vi "Prototype.vi"(8 "error in (no error)":errorcluster, 10 "Target Method Prototyper in":refnum<class "Target Method Icon Reader.lvclass">, 11 "Scripter in":refnum<class "Message Scripter.lvclass">) -> (0 "error out":errorcluster, 2 "Target Method Prototyper out":refnum<class "Target Method Icon Reader.lvclass">, 3 "Scripter out":refnum<class "Message Scripter.lvclass">)   [LabVIEW 2020, in "Message Maker.lvlib" / "Target Method Icon Reader.lvclass"]
uses:
  Target Method Icon Reader.lvclass
  Message Scripter/Message Scripter.lvclass
  Message Maker.lvlib
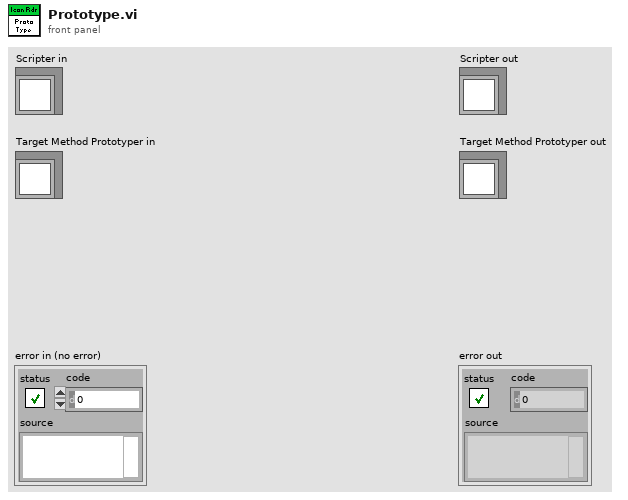
[diagram p1: front panel]
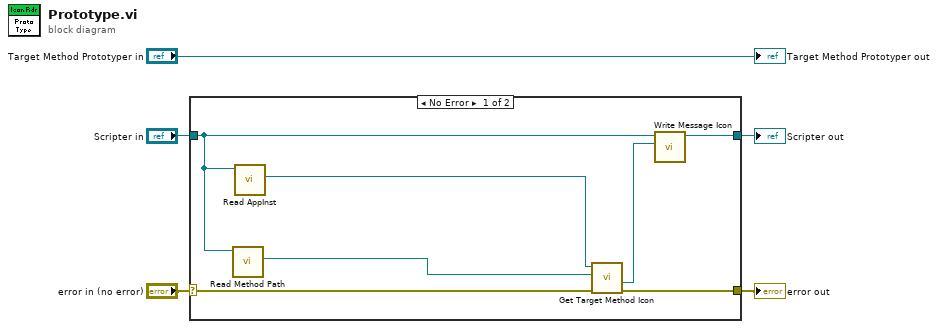
[diagram p0: block diagram]
diagram:
  n1 = case shown="No Error" "error in (no error)" {
    selector: "error in (no error)" -> [w12 w13]
    tunnel: "Scripter in" -> [w11 w14]
    tunnel: [w8 w14] -> w3
    tunnel: [w10 w13] -> w1
    frame No Error {
      n2 = call "Read Method Path.vi"("Message Maker in"=w11) -> ("Method Path"=w6:path)  [unwired: 10 in]
      n3 = call "Read AppInst.vi"("Message Maker in"=w11) -> ("AppInst"=w9:refnum<vi>)  [unwired: 10 in]
      n4 = call "Get Target Method Icon.vi"("error in (no error)"=w12, "Target Method path"=w6, "Application in"=w9) -> ("error out"=w10:errorcluster, "Icon out"=w7:refnum<class "Icon.lvclass">)  [unwired: 7 in]
      n5 = call-dynamic "Write Message Icon.vi"("Message Icon"=w7, "Message Scripter in"=w11) -> ("Message Scripter out"=w8:refnum<class "Message Scripter.lvclass">)  [unwired: 9 in]
    }
    frame Error {
    }
  }
  "error out" <- w1
  "Scripter out" <- w3
  "Target Method Prototyper out" <- "Target Method Prototyper in"
